vi "Find Version of Installed Driver Custom.vi"() -> ()   [LabVIEW 2014]
uses:
  <vilib>/nisyscfg/nisyscfg.lvlib
  <vilib>/nisyscfg/Close (System).vi
  <vilib>/nisyscfg/Get Installed Components.vi
  <vilib>/nisyscfg/Component Types.ctl
  <resource>/objmgr/nisysapi.rc
  <vilib>/nisyscfg/Component Type.ctl
  <vilib>/nisyscfg/Software 1.2.ctl
  <vilib>/nisyscfg/Resource Expert Info.ctl
panel:
  out "Array":bool[](array[boolean])
  out "ServiceType":u32[][](array[numeric])
  out "Experts":T1[][](array[typedef])
  out "Software Components":T2[](array[typedef]) {"component type" items=["standard", "hidden", "system", "unknown", "startup", "image"]}
  out "NI-Serial version":string
  out "NI-IMAQdx version":string
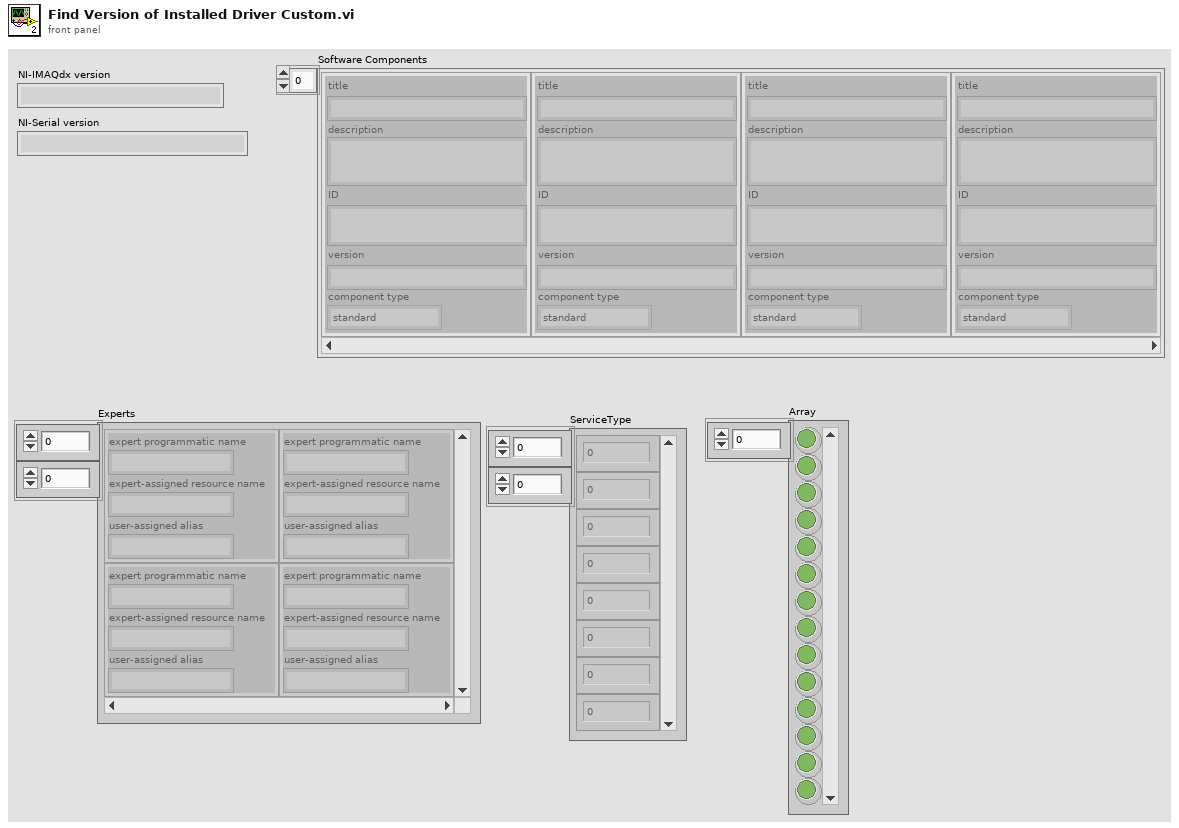
[diagram p1: front panel]
types:
  T1 = typedef "nisyscfg.lvlib/Resource Expert Info.ctl" = cluster{"expert programmatic name":string, "expert-assigned resource name":string, "user-assigned alias":string}
  T2 = typedef "nisyscfg.lvlib/Software 1.2.ctl" = cluster{"title":string, "description":string, "ID":string, "version":string, "component type":T3}
  T3 = typedef "nisyscfg.lvlib/Component Type.ctl" = u32
  T4 = typedef "nisyscfg.lvlib/Component Types.ctl" = u32
  T5 = typedef "Resource Expert Info.ctl" = cluster{"expert programmatic name":string, "expert-assigned resource name":string, "user-assigned alias":string}
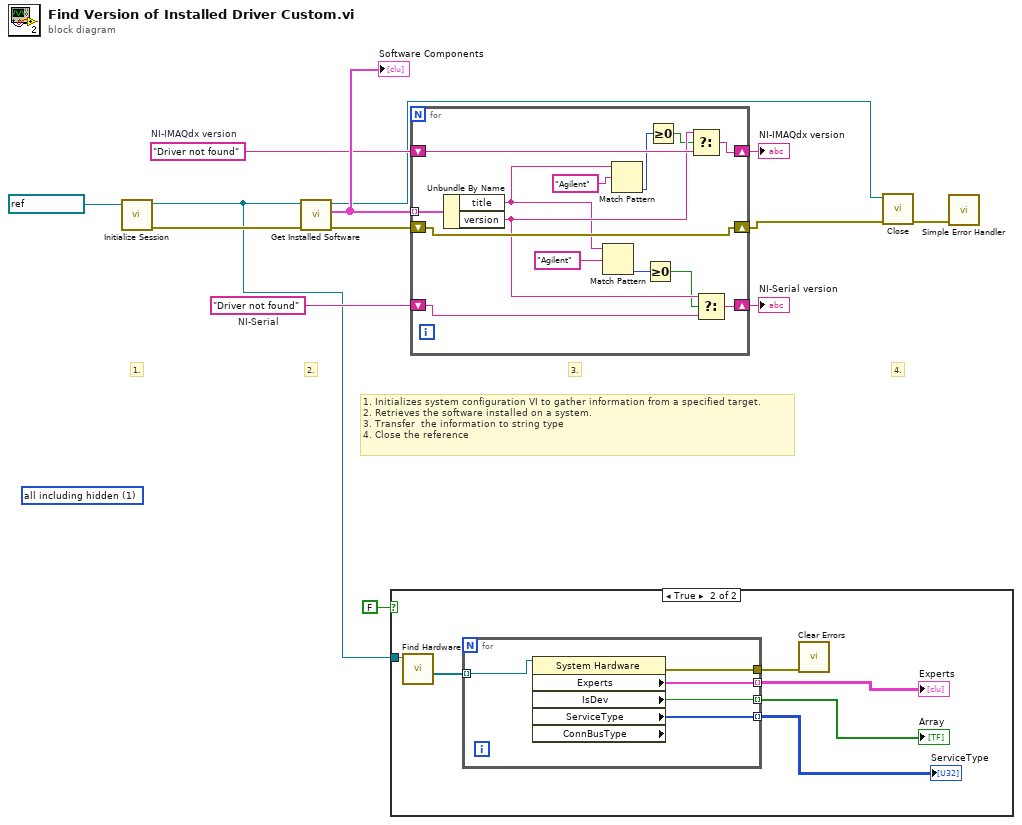
[diagram p0: block diagram]
diagram:
  (unwired) T4 1 items=["all visible", "all including hidden", "standard only", "startup only"] ("Item Types (all visible)")
  w11 = "Driver not found"  # NI-Serial
  w12 = "Driver not found"  # NI-IMAQdx version
  # "4."
  # "3."
  # "2."
  # "1. Initializes system configuration VI to gather information from a specified target.\n2. Retrieves the software installed on a system.\n3. Transfer  the information to string type \n4. Close the reference"
  # "1."
  n1 = call <vilib>:"Initialize Session.vi"("Target (localhost)"=refnum<k21> "localhost" ("session in")) -> ("error out"=w7:errorcluster, "Session out"=w1:refnum<k21>)  [unwired: 9 in]
  n2 = call-poly <vilib>:"Get Installed Software.vi"("error in (no error)"=w7, "Session in"=w1) -> ("error out"=w5:errorcluster, "Software Components"=w13:T2[], "Session out"=w6:refnum<k21>)  [unwired: 7 in]
  "Software Components" <- w13
  n3 = case shown="True" FALSE {
    tunnel: w1 -> [_ w17]
    frame False {
    }
    frame True {
      n4 = call <vilib>:"Find Hardware.vi"("Session in"=w17) -> ("Resources out"=w19:refnum<k20>[])  [unwired: 7 in, 3 out]
      n5 = for {
        tunnel: w19 -> [w24] mode=indexing
        tunnel: [w23] -> w18 mode=indexing
        tunnel: [w22] -> w15 mode=indexing
        tunnel: [w21] -> w16 mode=indexing
        tunnel: [w20] -> w14
        n6 = property class="System Hardware" props=["Experts", "IsDev", "ServiceType", "ConnBusType"](reference=w24) -> (error out=w20:errorcluster, "Experts"=w23:T5[], "IsDev"=w22:bool, "ServiceType"=w21:u32[])  [unwired: 1 in, 2 out]
      }
      "Experts" <- w18
      "ServiceType" <- w16
      "Array" <- w15
      n7 = call <vilib>:"Clear Errors.vi"("error in (no error)"=w14) -> ()  [unwired: 5 in, 2 out]
    }
  }
  n8 = for {
    tunnel: w13 -> [w38] mode=indexing
    shift-right: [w36] -> w10
    shift-left: w12 -> [w37]
    shift-right: [w34] -> w9
    shift-left: w11 -> [w35]
    shift-right: [w33] -> w4
    shift-left: w5 -> [w33]
    n9 = Unbundle By Name(w38) -> ("title"=w27:string, "version"=w32:string)
    n10 = Match Pattern(string=w27, regular expression="Agilent" ("y")) -> (offset past match=w30:i32)  [unwired: 1 in, 3 out]
    n11 = Match Pattern(string=w27, regular expression="Agilent" ("x")) -> (offset past match=w26:i32)  [unwired: 1 in, 3 out]
    n12 = Greater Or Equal To 0?(x=w30) -> (x >= 0?=w29:bool)
    n13 = Greater Or Equal To 0?(x=w26) -> (x >= 0?=w25:bool)
    n14 = Select(t=w32, s=w25, f=w37) -> (s? t:f=w36:string)
    n15 = Select(t=w32, s=w29, f=w35) -> (s? t:f=w34:string)
  }
  "NI-IMAQdx version" <- w10
  "NI-Serial version" <- w9
  n16 = call-poly <vilib>:"Close.vi"("error in (no error)"=w4, "Session in"=w6) -> ("error out"=w3:errorcluster)  [unwired: 9 in]
  n17 = call <vilib>:"Simple Error Handler.vi"("error in (no error)"=w3) -> ()  [unwired: 4 in, 5 out]
